vi "Left Join 2.vi"(9 "Array 2":string[][](array[string]), 11 "Array 1":string[][](array[string])) -> (2 "Left Joined Array":string[][](array[string]))   [LabVIEW 2020]
uses:
  a75eeadb-a20a-426b-b48b-c9c06ab4b909.vi
  965599a9-35c5-4084-8906-0a043779e57e.vi
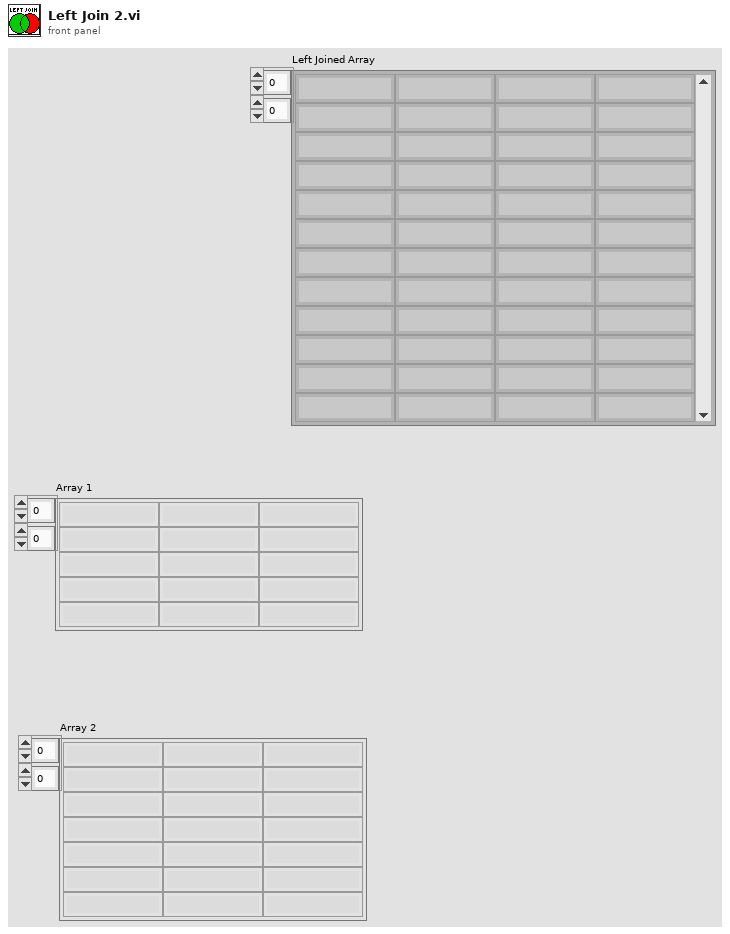
[diagram p1: front panel]
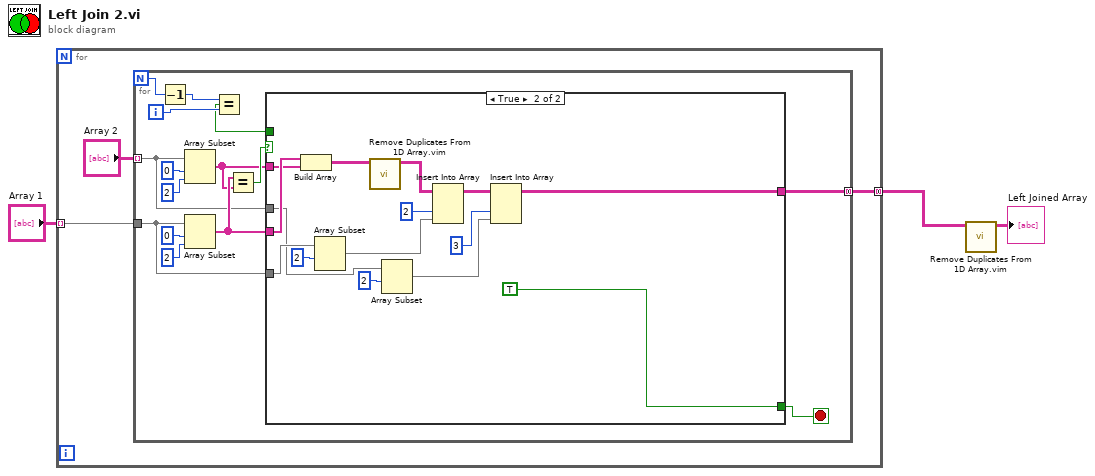
[diagram p0: block diagram]
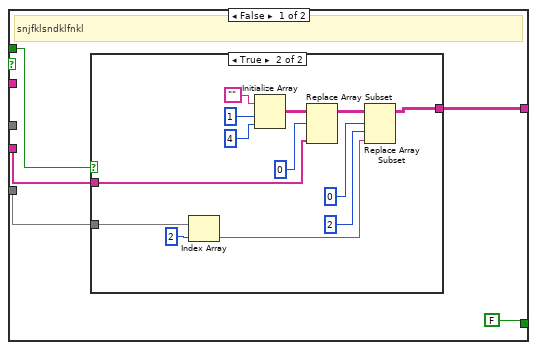
[diagram p2: hidden frame]
diagram:
  n1 = for {
    tunnel: "Array 1" -> [w5] mode=indexing
    tunnel: [w6] -> w2 mode=concatenating
    n2 = for {
      N -> [w8]
      tunnel: "Array 2" -> [w13] mode=indexing
      tunnel: w5 -> [w15]
      tunnel: [w20] -> w6 mode=concatenating
      i -> [w10]
      stop <- w11 stop-if-true
      n3 = Decrement(x=w8) -> (x-1=w7:i32)
      n4 = Array Subset(array=w13, index=0, length=2) -> (w12:string[])
      n5 = Array Subset(array=w15, index=0, length=2) -> (w14:string[])
      n6 = Equal?(x=w7, y=w10) -> (x = y?=w9:bool)
      n7 = Equal?(x=w14, y=w12) -> (x = y?=w21:bool)
      n8 = case shown="True" w21 {
        tunnel: [w24 w43] -> w20
        tunnel: w15 -> [w26 w50]
        tunnel: w13 -> [_ w47]
        tunnel: w14 -> [w25 w54]
        tunnel: w12 -> [_ w53]
        tunnel: [FALSE TRUE] -> w11
        tunnel: w9 -> [w22 _]
        frame False {
          # "snjfklsndklfnkl"
          n9 = case shown="True" w22 {
            tunnel: w26 -> [_ w38]
            tunnel: w25 -> [_ w30]
            tunnel: [_ w27] -> w24
            frame False {
            }
            frame True {
              n10 = Index Array(array=w38, index=2) -> (element=w35:string)
              n11 = Initialize Array("", 1 ("dimension size"), 4 ("dimension size")) -> (w31:string[][])
              n12 = Replace Array Subset(array=w31, new element=w30, index (row)=0) -> (w28:string[][])  [unwired: 1 in]
              n13 = Replace Array Subset(array=w28, new element=w35, index (row)=0 ("disabled index (row)"), index (col)=2 ("index (row)")) -> (w27:string[][])
            }
          }
        }
        frame True {
          n14 = Build Array(w54, w53) -> (w52:string[][])
          n15 = Array Subset(array=w50, index=2) -> (w49:string[])  [unwired: 1 in]
          n16 = call "Remove Duplicates From 1D Array.vim"("array"=w52) -> ("array with duplicates removed"=w51:string[][])  [unwired: 10 in]
          n17 = Array Subset(array=w47, index=2) -> (w44:string[])  [unwired: 1 in]
          n18 = Insert Into Array(array=w51, index (col)=2 ("index (row)"), new element=w49) -> (w45:string[][])  [unwired: 1 in]
          n19 = Insert Into Array(array=w45, index (col)=3 ("index (row)"), new element=w44) -> (w43:string[][])  [unwired: 1 in]
        }
      }
    }
  }
  n20 = call "Remove Duplicates From 1D Array.vim"("array"=w2) -> ("array with duplicates removed"=→"Left Joined Array":string[][])  [unwired: 10 in]
